vi "Check String Validity.vi"(6 "String Name for Error":string, 9 "Max Characters":i32=80, 10 "Valid String Specification":T1, 11 "String":string) -> (2 "string error":errorcluster, 3 "Valid":bool)   [LabVIEW 2015, in "NI_AWS_SQS.lvclass"]
uses:
  NI_AWS_SQS.lvclass
  Valid String Specification.ctl
  <vilib>/Utility/error.llb/Error Cluster From Error Code.vi
  <vilib>/ErrorRing/Error Ring.xnode
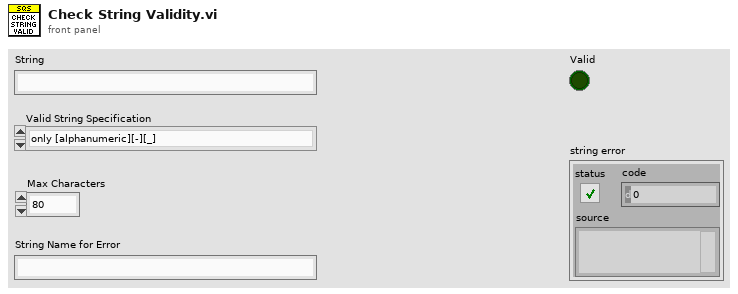
[diagram p1: front panel]
types:
  T1 = typedef "NI_AWS_SQS.lvclass/Valid String Specification.ctl" = enum16{"only [alphanumeric][-][_]"}
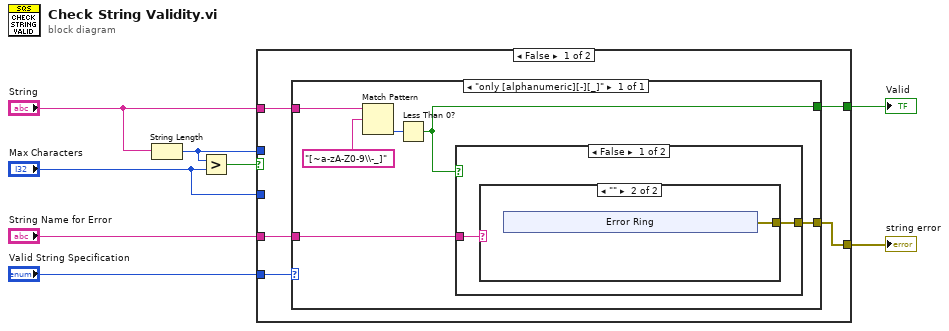
[diagram p0: block diagram]
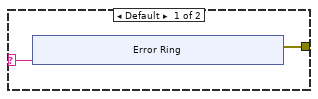
[diagram p2: hidden frame]
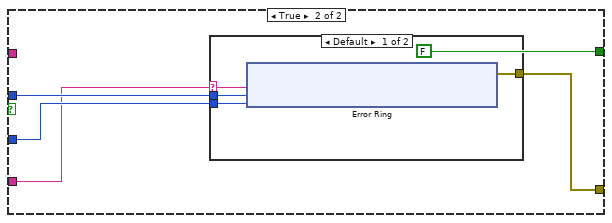
[diagram p4: hidden frame]
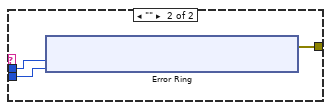
[diagram p5: hidden frame]
diagram:
  n1 = String Length(string="String") -> (length=w3:i32)
  n2 = Greater?(x=w3, y="Max Characters") -> (0:w8:bool)
  n3 = case shown="False" w8 {
    tunnel: "String Name for Error" -> [w10 w38]
    tunnel: "String" -> [w12 _]
    tunnel: [w11 FALSE] -> w5
    tunnel: "Max Characters" -> [_ w39]
    tunnel: w3 -> [_ w40]
    tunnel: [w9 w37] -> w2
    tunnel: "Valid String Specification" -> [w13 _]
    frame False {
      n4 = case shown="\"only [alphanumeric][-][_]\"" w13 {
        tunnel: w12 -> [w19]
        tunnel: [w14] -> w11
        tunnel: w10 -> [w16]
        tunnel: [w15] -> w9
        frame "only [alphanumeric][-][_]" {
          n5 = Match Pattern(string=w19, regular expression="[~a-zA-Z0-9\\-_]") -> (offset past match=w17:i32)  [unwired: 1 in, 3 out]
          n6 = Less Than 0?(x=w17) -> (x < 0?=w14:bool)
          n7 = case shown="False" w14 {
            tunnel: w16 -> [w21 _]
            tunnel: [w20 _] -> w15
            frame False {
              n8 = case shown="\"\"" w21 {
                selector: w21 -> [w23 _]
                tunnel: [w22 w31] -> w20
                frame Default {
                  n9 = xnode "Error Ring"("parameter 0"=w23) -> ("error out"=w22:errorcluster)
                }
                frame "" {
                  n10 = xnode "Error Ring"() -> ("error out"=w31:errorcluster)
                }
              }
            }
            frame True {
            }
          }
        }
      }
    }
    frame True {
      n11 = case shown="Default" w38 {
        selector: w38 -> [w43 _]
        tunnel: w40 -> [w45 w56]
        tunnel: w39 -> [w44 w55]
        tunnel: [w42 w57] -> w37
        frame Default {
          n12 = xnode "Error Ring"("parameter 0"=w43, "parameter 1"=w45, "parameter 2"=w44) -> ("error out"=w42:errorcluster)
        }
        frame "" {
          n13 = xnode "Error Ring"("parameter 0"=w56, "parameter 1"=w55) -> ("error out"=w57:errorcluster)
        }
      }
    }
  }
  "Valid" <- w5
  "string error" <- w2
